vi "VI_opener.vi"(8 "error in (no error)":errorcluster, 10 "vi_array_in":path[](array[path]), 11 "path":path) -> (0 "error out":errorcluster, 2 "vi_array_out":refnum<vi>[](array[refnum]))   [LabVIEW 2026]
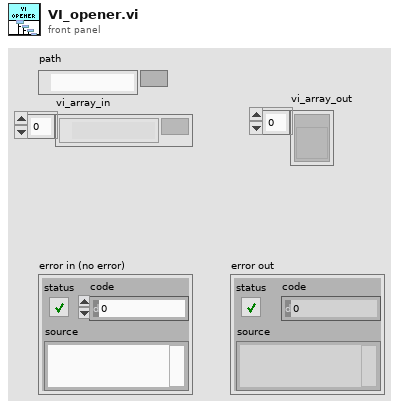
[diagram p1: front panel]
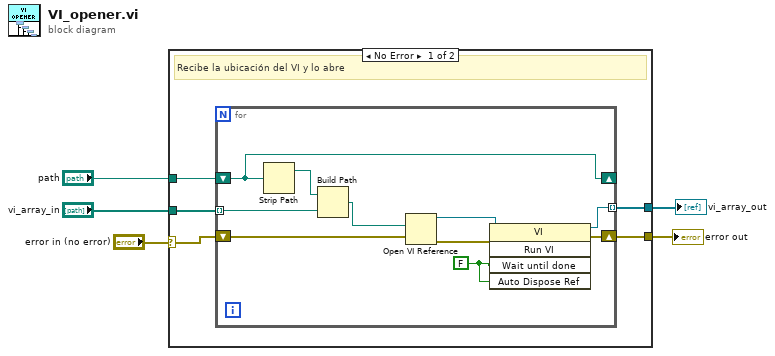
[diagram p0: block diagram]
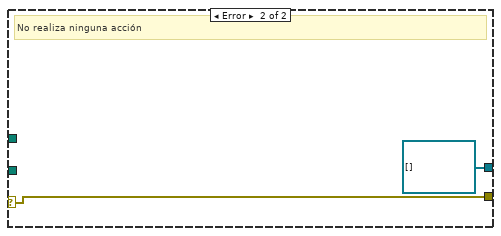
[diagram p2: hidden frame]
diagram:
  n1 = case shown="No Error" "error in (no error)" {
    selector: "error in (no error)" -> [w9 w22]
    tunnel: "path" -> [w10 _]
    tunnel: [w8 w22] -> w4
    tunnel: [w7 refnum<vi>[] []] -> w1
    tunnel: "vi_array_in" -> [w6 _]
    frame No Error {
      # "Recibe la ubicación del VI y lo abre"
      n2 = for {
        tunnel: [w14] -> w7 mode=indexing
        tunnel: w6 -> [w13] mode=indexing
        shift-right: [w15] -> w8
        shift-left: w9 -> [w16]
        shift-right: [w12] -> _
        shift-left: w10 -> [w12]
        w11 = FALSE ("Wait Until Done")
        n3 = Strip Path(path=w12) -> (stripped path=w18:path)  [unwired: 1 out]
        n4 = Build Path(base path=w18, name or relative path=w13) -> (appended path=w17:path)
        n5 = Open VI Reference(vi path=w17, error in (no error)=w16) -> (vi reference=w19:refnum<vi>, error out=w20:errorcluster)  [unwired: 4 in]
        n6 = invoke class="VI" method="Run VI"(reference=w19, error in=w20, "Wait until done"=w11, "Auto Dispose Ref"=w11) -> (reference out=w14:refnum<vi>, error out=w15:errorcluster)  [unwired: 1 in, 3 out]
      }
    }
    frame Error {
      # "No realiza ninguna acción"
    }
  }
  "error out" <- w4
  "vi_array_out" <- w1
